vi "power_supply.vi"(9 "byte count in":u32, 10 "write buffer in":string, 11 "VISA Refnum in":refnum<visa-resource-name>) -> (2 "return count 2":u32, 3 "read buffer 2":string)   [LabVIEW 2024]
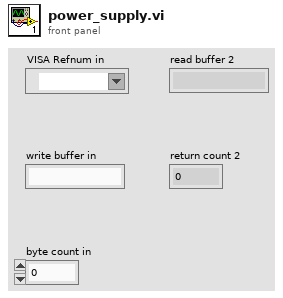
[diagram p1: front panel]
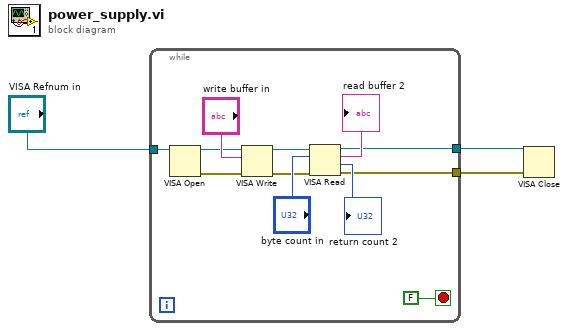
[diagram p0: block diagram]
diagram:
  n1 = while {
    tunnel: "VISA Refnum in" -> [w11]
    tunnel: [w5] -> w2
    tunnel: [w4] -> w1
    stop <- FALSE stop-if-true
    n2 = VISA Open(VISA resource name=w11) -> (VISA resource name=w7:refnum<visa-resource-name>, error out=w8:errorcluster)  [unwired: 4 in]
    n3 = VISA Write(VISA resource name=w7, write buffer="write buffer in", error in (no error)=w8) -> (VISA resource name out=w10:refnum<visa-resource-name>, error out=w9:errorcluster)  [unwired: 1 out]
    n4 = VISA Read(VISA resource name=w10, byte count="byte count in", error in (no error)=w9) -> (VISA resource name out=w4:refnum<visa-resource-name>, read buffer=→"read buffer 2":string, return count=→"return count 2":u32, error out=w5:errorcluster)
  }
  n5 = VISA Close(VISA resource name=w1, error in (no error)=w2) -> ()  [unwired: 1 out]
